vi "Project Test 2.vi"() -> ()   [LabVIEW 2022 SP3]
panel:
  out "Warning Lights":bool[](array[boolean])
  in  "STOP":bool
  out "Boom gate closed if ≠ 0":dbl
  in  "Sensor 2":bool
  in  "Sensor 1":bool
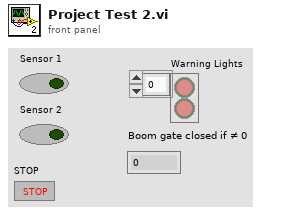
[diagram p1: front panel]
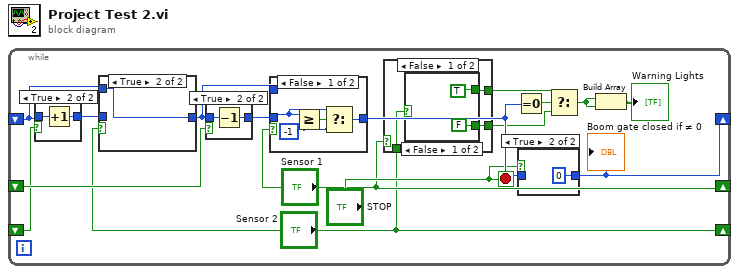
[diagram p0: block diagram]
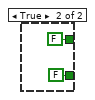
[diagram p2: hidden frame]
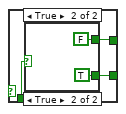
[diagram p3: hidden frame]
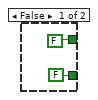
[diagram p4: hidden frame]
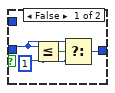
[diagram p5: hidden frame]
diagram:
  n1 = while {
    shift-right: ["Sensor 1"] -> _
    shift-left: _ -> [w12]
    shift-right: [w10] -> _
    shift-left: _ -> [w8]
    shift-right: ["Sensor 2"] -> _
    shift-left: _ -> [w11]
    stop <- "STOP" stop-if-true
    n2 = case shown="True" w11 {
      tunnel: [w36 w38] -> w9
      tunnel: w8 -> [w36 w37]
      frame False {
      }
      frame True {
        n3 = Increment(x=w37) -> (x+1=w38:i32)
      }
    }
    n4 = case shown="True" "Sensor 2" {
      tunnel: [w33 w35] -> w7
      tunnel: w9 -> [w32 _]
      tunnel: w8 -> [_ w35]
      frame False {
        w31 = 1
        n5 = Less Or Equal?(x=w32, y=w31) -> (x <= y?=w34:bool)
        n6 = Select(t=w32, s=w34, f=w31) -> (s? t:f=w33:i32)
      }
      frame True {
      }
    }
    n7 = case shown="True" w12 {
      tunnel: [w44 w46] -> w13
      tunnel: w7 -> [w44 w45]
      frame False {
      }
      frame True {
        n8 = Decrement(x=w45) -> (x-1=w46:i32)
      }
    }
    n9 = case shown="False" "Sensor 1" {
      tunnel: [w41 w43] -> w6
      tunnel: w13 -> [w40 _]
      tunnel: w7 -> [_ w43]
      frame False {
        w39 = -1
        n10 = Greater Or Equal?(x=w40, y=w39) -> (x >= y?=w42:bool)
        n11 = Select(t=w40, s=w42, f=w39) -> (s? t:f=w41:i32)
      }
      frame True {
      }
    }
    n12 = case shown="False" "Sensor 1" {
      tunnel: "Sensor 2" -> [w17 w26]
      tunnel: [w18 w25] -> w2
      tunnel: [w19 w24] -> w1
      frame False {
        n13 = case shown="False" w17 {
          tunnel: [TRUE FALSE] -> w18
          tunnel: [FALSE FALSE] -> w19
          frame False {
          }
          frame True {
          }
        }
      }
      frame True {
        n14 = case shown="True" w26 {
          tunnel: [FALSE FALSE] -> w25
          tunnel: [FALSE TRUE] -> w24
          frame False {
          }
          frame True {
          }
        }
      }
    }
    n15 = Equal To 0?(x=w6) -> (x = 0?=w16:bool)
    n16 = case shown="True" "STOP" {
      tunnel: [w47 0] -> w10
      tunnel: w6 -> [w47 _]
      frame False {
      }
      frame True {
      }
    }
    "Boom gate closed if ≠ 0" <- w10
    n17 = Select(t=w2, s=w16, f=w1) -> (s? t:f=w14:bool)
    n18 = Build Array(w14, w14) -> (→"Warning Lights":bool[])
  }
